vi "Main_GOOP4_CreateObjects_Open_GDS.vi"() -> ()   [LabVIEW 2019]
doc: "This is the main VI for the Project \"GOOP4_CreateObjects_Open_GDS.lvproj\""
uses:
  GOOP4_Sub_class/GOOP4_Sub.lvclass
  GOOP4_Base_class/GOOP4_Base.lvclass
  Interface by vi server_Interface/Interface by vi server.lvclass
panel:
  out "error out":errorcluster
  out "Str":string
  out "i":i32
  out "Sub i 2":i32
  out "Sub Str":string
  out "Sub error out":errorcluster
  out "Base error out":errorcluster
  out "Sub i 1":i32
  out "Base i 2":i32
  out "Base i 1":i32
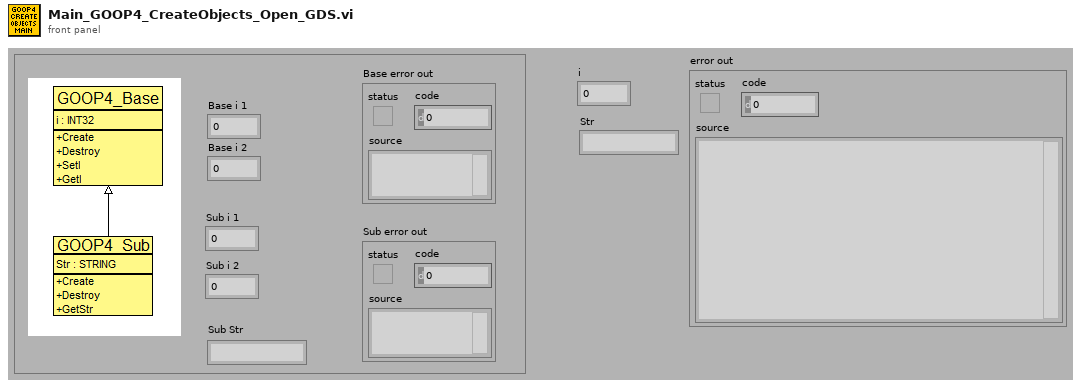
[diagram p1: front panel]
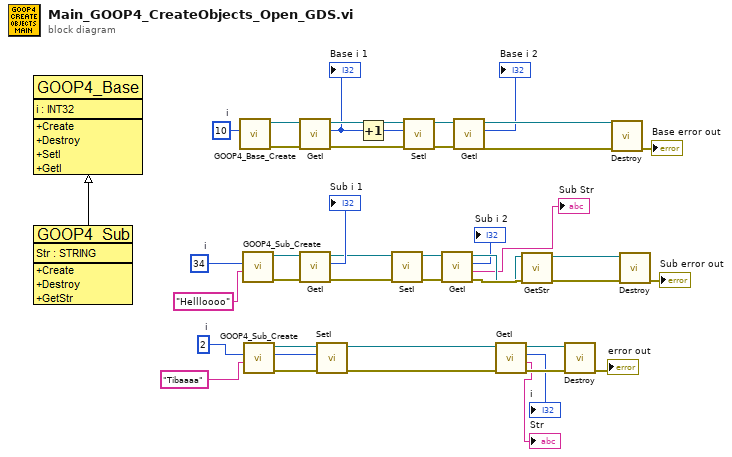
[diagram p0: block diagram]
diagram:
  w1 = 2  # i
  w28 = 34  # i
  w36 = 10  # i
  n1 = call "GOOP4_Base_Create.vi"("i"=w36) -> ("error out"=w34:errorcluster, "reference out"=w35:refnum<class "GOOP4_Base.lvclass">)  [unwired: 9 in]
  n2 = call "GOOP4_Sub_Create.vi"("Str"="Hellloooo", "i"=w28) -> ("error out"=w26:errorcluster, "reference out"=w25:refnum<class "GOOP4_Sub.lvclass">)  [unwired: 8 in]
  n3 = call "GOOP4_Sub_Create.vi"("Str"="Tibaaaa", "i"=w1) -> ("error out"=w9:errorcluster, "reference out"=w10:refnum<class "GOOP4_Sub.lvclass">)  [unwired: 8 in]
  n4 = call-dynamic "GetI.vi"("error in (no error)"=w34, "reference in"=w35) -> ("error out"=w32:errorcluster, "i"=w31:i32, "reference out"=w33:refnum<class "GOOP4_Base.lvclass">)  [unwired: 6 in, 1 out]
  "Base i 1" <- w31
  n5 = call-dynamic "GetI.vi"("error in (no error)"=w26, "reference in"=w25) -> ("error out"=w19:errorcluster, "i"=→"Sub i 1":i32, "reference in"=w14:refnum<class "GOOP4_Sub.lvclass">)  [unwired: 6 in, 1 out]
  n6 = call "SetI.vi"("error in (no error)"=w9, "i"=w1, "Interface In"=w10) -> ("error out"=w3:errorcluster, "Interface Out"=w8:refnum<class "GOOP4_Sub.lvclass">)  [unwired: 7 in]
  n7 = Increment(x=w31) -> (x+1=w30:i32)
  n8 = call-dynamic "SetI.vi"("error in (no error)"=w19, "reference in"=w14) -> ("error out"=w12:errorcluster, "reference in"=w13:refnum<class "GOOP4_Sub.lvclass">)  [unwired: 8 in]
  n9 = call-dynamic "SetI.vi"("error in (no error)"=w32, "i"=w30, "reference in"=w33) -> ("error out"=w40:errorcluster, "reference out"=w39:refnum<class "GOOP4_Base.lvclass">)  [unwired: 7 in]
  n10 = call-dynamic "GetI.vi"("error in (no error)"=w12, "reference in"=w13) -> ("error out"=w18:errorcluster, "Str"=→"Sub Str":string, "i"=→"Sub i 2":i32, "reference in"=w17:refnum<class "GOOP4_Sub.lvclass">)  [unwired: 6 in]
  n11 = call-dynamic "GetI.vi"("error in (no error)"=w40, "reference in"=w39) -> ("error out"=w37:errorcluster, "i"=→"Base i 2":i32, "reference out"=w38:refnum<class "GOOP4_Base.lvclass">)  [unwired: 6 in, 1 out]
  n12 = call "GetI.vi"("error in (no error)"=w3, "Interface In"=w8) -> ("error out"=w6:errorcluster, "Str"=→"Str":string, "i"=→"i":i32, "Interface Out"=w7:refnum<class "GOOP4_Sub.lvclass">)  [unwired: 6 in]
  n13 = call-dynamic "GetStr.vi"("error in (no error)"=w18, "reference in"=w17) -> ("error out"=w23:errorcluster, "reference in"=w24:refnum<class "GOOP4_Sub.lvclass">)  [unwired: 7 in, 1 out]
  n14 = call-dynamic "Destroy.vi"("error in (no error)"=w6, "reference in"=w7) -> ("error out"=→"error out":errorcluster)  [unwired: 8 in, 1 out]
  n15 = call-dynamic "Destroy.vi"("error in (no error)"=w37, "reference in"=w38) -> ("error out"=→"Base error out":errorcluster)  [unwired: 8 in, 1 out]
  n16 = call-dynamic "Destroy.vi"("error in (no error)"=w23, "reference in"=w24) -> ("error out"=→"Sub error out":errorcluster)  [unwired: 8 in, 1 out]
